vi "Main_14b.vi"() -> ()   [LabVIEW 2023]
uses:
  ENUM_Type.ctl
  <vilib>/Utility/miscctls.llb/LVMapReplaceAction.ctl
panel:
  out "Repeat index":i32
  out "Firt Index":i32
  out "Answer 2":i32
  out "Start":T1[][](array[typedef])
  in  "Puzzle":string="O.OO.#...#.O#...#...O..O.#O..O.##.....###O.O##O.O....OO.....##..##.#..O#.........O#..#..O...#O.....O\n.....###.O....#.#O.....##..O##O.......##......O..#..##.#.O#...O...O.O....#.###O.OO#.#O.#.#..O..OOO..\nOO......#.#..##O........O.###..#.#........O#..O....O#.#.##.OO.....O#.........###O......#..#.O..#....\n..#O...O....#.#.#O#....#.O#....OO.OO.O#...O##.O........O.#O.OO.O.....O.#.O.#....O.....O..OO.OO...O.#\n..#O...#.....O#O...###O......O#.##O..O#.O.O.#..#O#.O....O..O#...OO...O..#.O.......O.##OO.#...#...##.\n.#......O.OO#....O#O#OO.O..O......OOO..O....O....#OO....O...#.O.O.O..O...OOOO...#......O..#O..#O....\n..O.#.O.#..OO...........#..#......#.#...#...O...#...#...O##..O..#..O.#...O..#.O...#....#..OO..O..#.#\n.##..O..##O......#...##....#..#..O....#..##.#.O#....O#..#...O.O....O.O.........OO.#.OO......O.......\n..##O.O...O.O..O##OO..#.O..O.#...O..#..#.O...O....##...#O...O......#.....O##O#..O.#..#..O...#...#.O.\nO..##...##...#.#.OO#...OO#O..O...O.#O..#.O......O##......#O..O..OOOOOO..O.##.O...#O.....O##......OO.\n.........O..O#.....#...#......OO###OO.O.O#...#.O....O..##..O#.....O.#.##O.#......#.O.....OO#.#..##O.\nOO#O...#...OO.O####.OO.#.#.......O......O#..O#..#...#O....#.....OO#O......#O#...O#.OO......O....O#..\n.O.........#.#O#....#OO..#.........OO....O...#.O.O.O.OOO.O..O.....O.#....OOOO....OO.......#.#.O.##..\n....#.....#.O.#O...O#OO#...##.#.#..O.O.O....#O.#.#.O...#O#O.O#O...O..#OO..O###.OO..#.....OOO.#......\n#OOO..OO.O.O..O..O....#....O..O.#...O...O...##.O##..O...OOOOO#.........OOO##..#...OO#O#O.....O...##.\n.......O#..#OO.O.O..OO.O#..O.......##....OO#.O..O..O#...#..#...O.##.....#..........#.....#.O...#...O\n......O.#.O...O.......O#..O..OOO#...#........###.O..#....O.O#.OO.O..#.O#O.O.O.......O.##.OO......O.#\nO....O..........#....##.###..#...O#.O..O.##.O....O..O..O..##.O.O#OO...O.#.O##..#.#.......#.O..O..O.O\n..O#..O.#.##..O#..O#..O..O..O....OO...O##..#...O.OO..#.#.#.###O.O...#O.##..#.....#..#O.O.O...#O.O#..\n..O.##........OO.....OO.O..#.....OO.O..#...#..OOO..#....#....#.OO.#.#........OO...O.#O....##O..OOOO#\n.........#.#.OO.#O...#...O#........O..#.#........O......O#.OO..#..#....O##OO.......O..O.O.O.........\n#..O..#..OO.O.O....O..O.O.#.O.O#O...O.OO..#......OO.#..O....#.....#OOO#.OO#.OO........###....O.....O\n..O..O.O.O.....O..#.O..##.O..##..O###........O.O..#...O....OOO#.OO.#O...O..##....#.#O...#..O...O...#\nO#...O..O.#.#......O..O.#OO.....O..#.......O.##O........#O.OO..#..O.##..O.#...O...#O.....#.#..OO##..\nO.OO..O....O.#..O##O.#.O.O#O..##...O..##...#.O#.....O##.#O..O.O.....O....##..O.###......#........O..\n.....##.#.......O.OO....#..##............##..O..#.......O..O..#.O...O#..O.O.##..O..OO.O.....O...O...\n##.O.#....O..OO..OOO.OO.##..OO.OO.#...O#.....#...##...O#....OO..O.O...O...O.#....OO...#..#O#.##..#..\n........OOO....O...#.O...O..#......O....#O#.#O...O#.O........O.O...OO#....O..#.#.#O.O...OO....O.#O..\nOO...O...O..#.OO..O#.OO###..O.......#..O..O.####O....O.O.O#O.#..O..##OO..O..#....#..O#O....#..O...O.\n..O....#.O.O....O...#.........#..O#.#..OO....#...##.OO..OO.O...OOO..O..O#.###.......O#...#....OO...#\n.O...OO.O.O...#.......#.O.O.....O...OOOO.#O.O..O..OOO.OO...............#O...##O..OOO##....#O.O#.##..\nO....O...O.#...........#..#.#OO###O.O...#.O#..O.....O...O....O...#...O.OOO.OO#..OO...#..OOOO...#..#.\n....O...OO.#.O...O..#....O.O.#O..O....O..O..##O.#O....O..O.....O.......OO.......#OO#.##.O.#.O..#.##O\n#OO#.#....###O#..OO..#..O.......O.O...OO#.#O.....O.O##.O...#.##O#...O#......#..#..O#O.O.....OO.O#.O.\n...O#....O...O......#..O#O..OO.O#.OO.#.......#...O..O.....O.#O..O..O.....#OO#.O..#....#O.#O..#......\n..O.....O.......#O....O#...##.....#..O.#....#.#.#O#.#....O....#..O.O......OO....O.#OO#OO.....O......\n.#..O..#..O##...#O.#.##O#.#.#O....O#..###.OO..##..#..........O#O.#..#....O...##.......O.O.O##O#..#O.\n.#.....O..O.#..#..O....O...#.....#O.O.....OO.#..#......##........O.#.#......#...OO#....O#O.....#..O#\n#.....O.....O...O..##O.OO#OO......O#..O......O...O...#.....OO..#...O..#.....##.#.O...#..#O......OO.O\n.#..#.#.#...O#.......#.O....O..#.#.#.....O...................#.O...OOO#.....O.O.....O..O.#.....#.O.O\nO....O.....O.....O#O...O.O.O#O.#O..OO#OO..#OO.OO##.....##O#.O.O..#.....O..OO.##.#.......#...O..OO.O.\n.O#..O..#....##......O....#.#.#......#........##...#....#.......#.....O......##.#.....O.O....OO#.O..\n....OO.OO#...O..#O#O.#.O.#..OO...OOO...#O.#..#..#.#O...#O.#.O..##..O.##..O#.#.....#..O...#.O...O#.O#\n....O#....O.O#OOO...#.#.........O.O....#..O...#...#.....O.O.O.O....#.OO.##O.....#.#.#.#O..O#.O.#.OOO\nO#OO..O.#.......###..OO..O........O.##O.#O##..O...O.#OO.....#...O......O.OO...O..OO....O..O..#.#...O\n.#.O.O.O.#......O......##O...OO.....O....O#.....O#....#.......#O..#...##..O..#O.O.O..O....O.........\n...#.........OO..O.O#..O.#....#...OO##...O..OO.......#.#OO..#...#..##.#...OO#...#O.#...O.....O...#..\n#.....#O......O....O#.....#.#O.OO..........O.O...#....#.###O.O..O...#...#..#....O..O..O#.O.........#\nO.O.O...O...#.....#.#....O.O.O.....OO....#..OOO......O.O.......O#O...#.#O##O.####.........O#O.......\nO.O...........O#...OO..#O.O.O......O.......##.O...O..##...O.#OO...#OO...#...#O#.##O.#......O.##....O\nO..#...........O..O......OOO....#....OO.O...#O..O.O#......#...........#O...#O..O....#.#.#..#...#O...\n..O.....#...#...O.#.O..##.........O#..##.....#O.........................##...#.#..#.OO#O...#OOO#O.##\nOO..O.O.....O#.O....O##...O.O#.OO.#..O.....O...##.O#..O......OO..#..O.....##.....OO#OO...#O......O.O\n.OO...#....#O..#.....OO..O.O.......O#...O#..O#..#.O....#.O.#.O...O.#.O.#...#..OO.......O#....OO..O..\nO.OO..#.OOO.#.O#...#.#..O..O#.#.#.#.....#.O#..O....O..OO...O..#..#....OO#O.#......O#..##...O...O.#O.\n....#....#...OO#...O.O#OO.#.#OOO..O...OO.O..#.O#..#..O.O..#.#........OO#O.#.#.#.....OO......##.#.O..\n.#.O.OOO#OOO...##O#.#...#...##O.#...O.......###O#.##..O#..#.##...O..O.O.........O..#..O##......#.##.\nO...#..#....#O..##..O.O##..O.O###O.......O...#.O#.O#..O...#.#.O..#.....#.....O..O..OOO.OOO..O..OOO..\n...O#.O....O.O.#.O..#.O..####...OO......#OO....O#....O..O...O...OO..OO.OOO#....#..#.O.O..#..#.....O.\nO.O##O.O.O.#.O.#........#O......#O.##...##OO.......O#..#..#.O....OO........#.#O..#O.........OO.O#..O\n.......#.....O...O.O.#O##.O.OO#.....O.O#O....O.#.##.#.......##.O.O.###O...O.O#O##...#...#...O..#....\n.O#...#O...#....O##.O..........O.O.#..O.O..OOOOO.......OO.O#...O...O...#O###OOO.#OOO..............O#\nO.#.#.......OO..OO.#.O#.....#.O#O...#......O....O...O.O.....OO.#O.......#..O...O.....##OO#.....OO#.#\n...O#...#.....#..#O.#..O..O.#O#O.#...OO#O.O....O.#...#O#O....#......O..#O...#....O..O.O........#..#.\n.O.......#..O#...O....................#.##O......#.#......####..OO#...OO.##..#........#.OO..#OOO.###\n......O...O..O##.......O...O##O.O....#..#.##...#OO..##..........#..............##O.......O...#O###O.\n.........#..OO.#.......OO...O....#O.#.......O..##...###..O...#OO.O.O...#...#OO....##O.....#O.O..#...\n..#....O..O......#.#....OO#....#...O.#.OO.O#.....O#.#......O.#O.........O....O....#..O.........O....\n.OO.......#.....O.O..O#....O.#.....O..O#O...O#.....OOO....##..O.O..O#.OO...#....#...O..#..##..#..#.O\nO..#..OO##.#..OOO..#...#.OOO..O..##..O..##O.......O.O..O...#.O...#..###.#.#.#...#O..O......#.O#....#\n...O..#O..O..OO.#....#...##...O...#.......OOOO#...O.###.O.......#O.O#.##.##O..#...O...O.O..#....OO..\nOO.........OO...O.O............O....O.O...O.O.O.......O.OOO.O#....#O.O..#.....O#...#...#....#......O\n#.OO#........OO..#OO.....O.#...#..#O.O...O.....#..O.......O...O..O...O.O.O....##...O....O.OO.....#.O\n..O....#..O....O#.....#..#O......O......#...#O.......O.O...##O.#...O#..O#.#O###...#.OOO.#O...O#....O\n.#.#..OO.#..O###....O.#......O..OO...O.O..O.#.O....O.#..O.....O#....O....#.......O.O...O......OOO.#.\n...OO#.OO#O....O....O.O.#.O.#O..#.O#...###...#......#...OO##.#.#..O#...#....#.#.#.OO....O...OOOO...O\n..O.#..O...O...O#O......##.....O...O..O....#....O..#OO.#.O......#O.OOO.O.O..#........##...#O.#O...O.\n..O.OO.....O...#..O..#...O...O..#O..O#..##.....#....#.#O.#.......#O##....O.OOOOOOOO#.O...O.O#..#O##.\nO.OO.####..OO...OO.O........OO#.O.O...#....#..OO......O.O...O..#.##....O....O......#O........#O.O#..\n.#O.#...#.#...OO#.O.#O.....O##.O.OO.O..#..#O.....O...#.O.O#.....###.....#O.O.......O.#O.O#..#.O..#..\n.O......O........O...#O....##.....#O..OO.O..#.....O.#..O...#O#.#..##.#O..........O.O.O..#....#..#..#\n.OOO..O...#O.O#..#....O......O.O...O#O.....#..OO......OO.#O..O..O###......O.#.#.#.O....#...O........\n.##.....#OO#.##.....#....O..O.....OO..OO##...O...O#.##.OO#....#.......#...O.O.#.O........OO...OO....\n......OO#.....OO#OO......#.O....##..O.O#...O....#..O.O.#O.#...#.O..#.O.O#O....O.O..O.O.O.#OO.##.OO.#\n.O..OO##....O###......####.OO...O#..#..##.##.O..#..##OOO...#..#O##.#..#........#...#....O.......#.OO\n..O..O.O..#....#.#O.#.#OOO....O.##.....OO....#..O...#...#O.........O....O..#..........#.O..O.OO.O##O\nOO.......#...O#.#.......O...O.OO#.O.O.....O.....#...##..#....#.......O#.#O..O.O.......##...OO..#O...\n#O#....#.#.O..#...OO...##.#.#.O#O#...#........O..OO..#..O#..O..O.O.#O...#.....#O.#O.O#..OOO#.O.O..#.\n.#O...OO.##.#.....O...O#O................O.O..O#...#..O.#OO..O....OO...O.#...O#.#.O...O#....OO#.#...\nO#...###.OO.O...O.O#O#..O.O...O.#.....O......O...#...O.O....#...O...O#.#...##....O...........#O...#.\n.....#OO.#.OO...##.O....#OO#.....O..##...OO#.......O...##..#....#..#..##.#O.O##..O.#.O.#.O#OO.O.#.#O\nO##.#..O.OO..O.O.OOO.O...O..O.O..O.O.O..#.........#.....OO.#.......O#....#.......#O.#.O..#...O#..OOO\n.#....O.O..O##...#.OO#.O#..#OO..O.#...O....##.#O.O#O#...#.........O.#..#....OO..O.#........##O.##O..\n.....#....OO#...#.OO.O.O....O..#O.#.O#.O##.O..#.#O.#..O.#.O..O#.#.O.O.O#O....OO#...O......OO#..OO#O.\nO..O.#O..OOO..O...O...#.......#O.OO....O..#...O.....O.#.OO....#.O.OO...O#...OOO###.O..#.....O..O#.#.\n.OO......O#O.......OOO.......O..O...........O..##.....OO..##...O.O.O...O.O.O.....O..OO..O#....#.O..#\nO....#....#O.####.O...#....O....#O..#O...O.O....O.O#..O.........O#.......O....O..O...#.##..O.OO.OO..\n.O###O...#OO.OO........O.O#.O.O....O.O...##.O#..###..........#..O#.O..O.OO.O..#O#OO..O#.O.##.O.OOO##\n#.#O#..O.#...O#..#.......O#..#...#...#O..#.O.....O...O.......#O.#...#OO.O....OO..O...#.#....#O......\n..O.#O.O.O#..#.O...#.....#..O..##..O......O.OO.O.###.....#.O..O...OO#.OO.....#...OO#O..#..#O#...O..O"
  in  "Example":string="O....#....\nO.OO#....#\n.....##...\nOO.#O....O\n.O.....O#.\nO.#..O.#.#\n..O..#O..O\n.......O..\n#....###..\n#OO..#...."
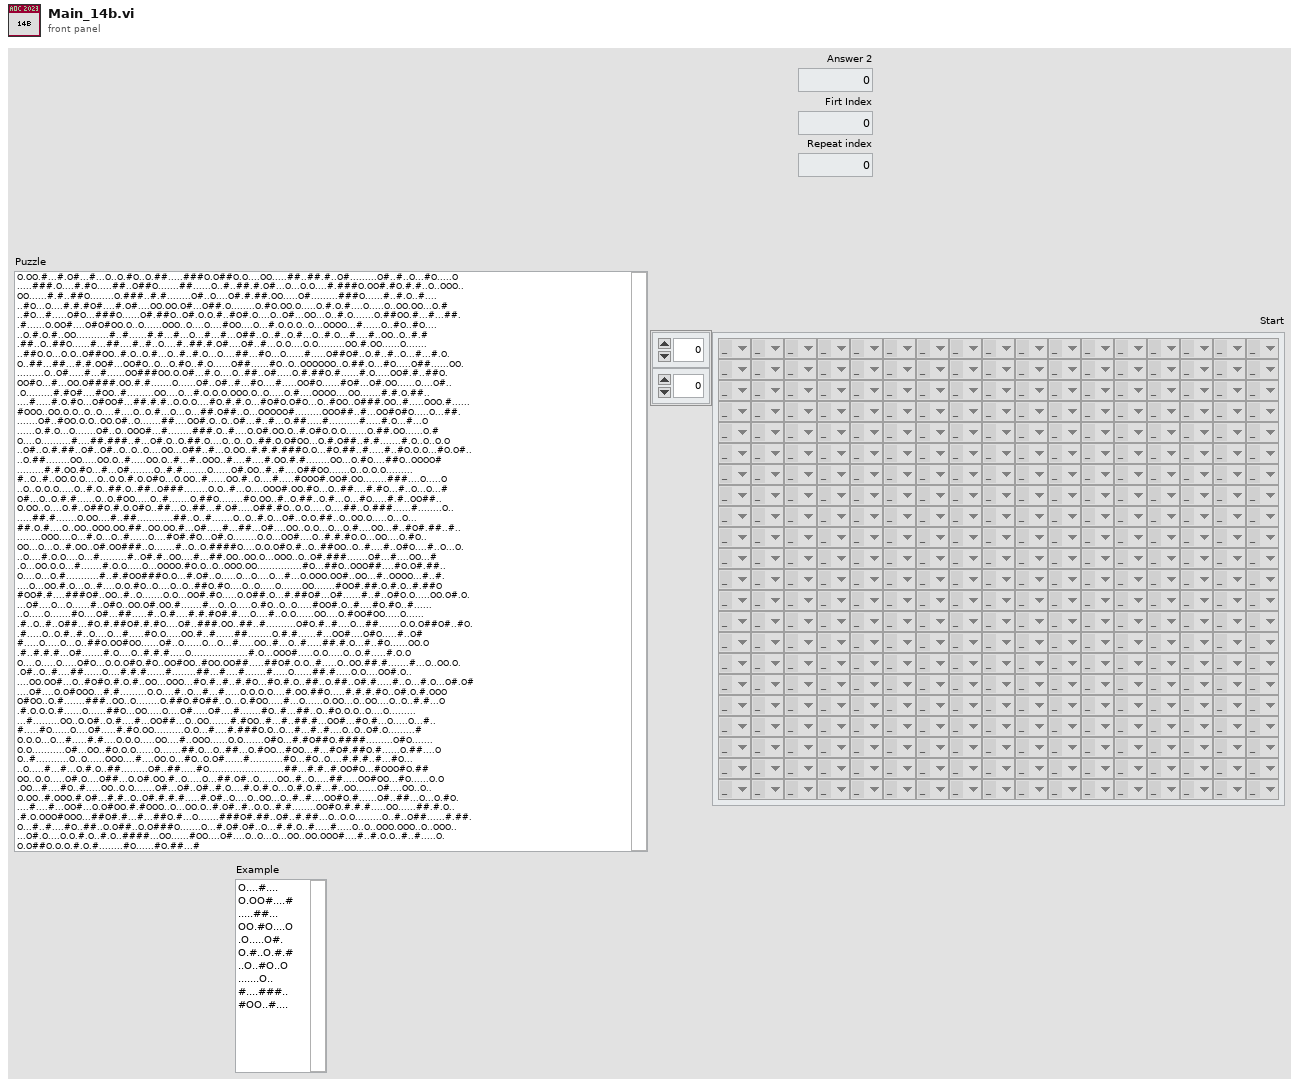
[diagram p1: front panel]
types:
  T1 = typedef "ENUM_Type.ctl" = enum16{"_", "O", "#"}
  T2 = typedef "LVMapReplaceAction.ctl" = enum32{"Modify Entry only if found", "Add or Modify Entry", "Delete Entry"}
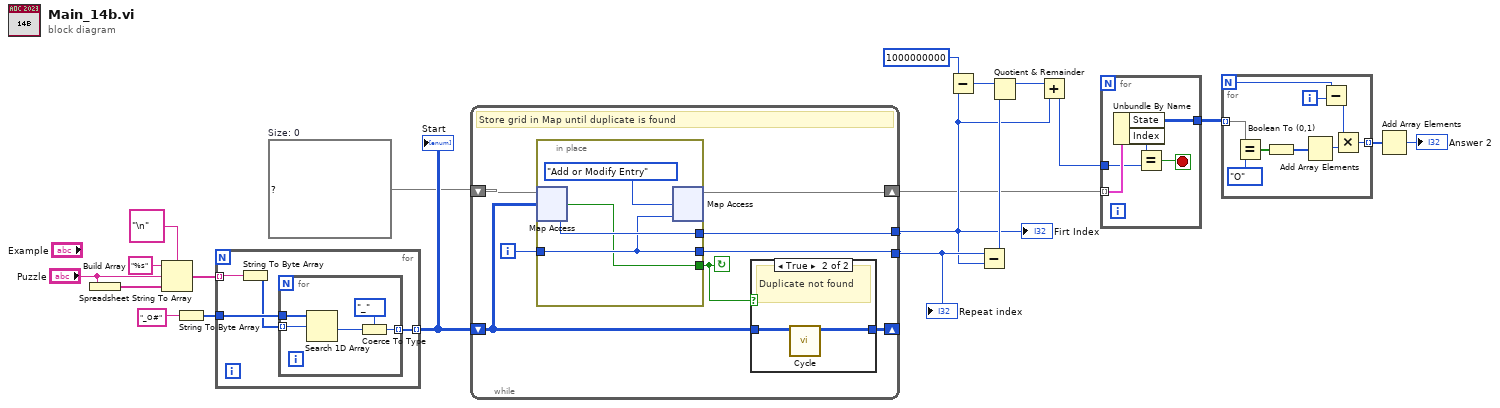
[diagram p0: block diagram]
diagram:
  w13 = map{T1[][], i32} {}  # Size: 0
  n1 = Build Array("Puzzle") -> (w20:string[])
  n2 = Spreadsheet String To Array(delimiter (Tab)="\n", format string="%s", spreadsheet string="Puzzle", array type (2D Dbl)=w20) -> (array=w17:string[])
  n3 = String To Byte Array(string="_O#") -> (unsigned byte array=w15:u8[])
  n4 = for {
    tunnel: w17 -> [w24] mode=indexing
    tunnel: w15 -> [w23]
    tunnel: [w21] -> w14 mode=indexing
    n5 = String To Byte Array(string=w24) -> (unsigned byte array=w22:u8[])
    n6 = for {
      tunnel: w23 -> [w29]
      tunnel: w22 -> [w28] mode=indexing
      tunnel: [w25] -> w21 mode=indexing
      n7 = Search 1D Array(1D array=w29, element=w28) -> (index of element=w27:i32)  [unwired: 1 in]
      n8 = Coerce To Type(0:w27, 1:ENUM_Type."_" ("Enum")) -> (2:w25:T1)
    }
  }
  "Start" <- w14
  n9 = while {
    shift-right: [w37] -> _
    shift-left: w14 -> [w35]
    shift-right: [w31] -> w6
    shift-left: w13 -> [w36]
    tunnel: [w32] -> w7
    tunnel: [w30] -> w10
    i -> [w34]
    stop <- w33 continue-if-true
    # "Store grid in Map until duplicate is found"
    n10 = in-place {
      in-place-border: w34 -> [w42]
      in-place-border: [w41] -> w33
      in-place-border: [w43] -> w32
      in-place-border: [w42] -> w30
      n11 = in-place-map #1(w36, w35) -> (w43:i32, w41:bool)  [unwired: 1 in]
      n12 = in-place-map #1(w42, LVMapReplaceAction."Add or Modify Entry" ("action")) -> (w31:map{T1[][], i32})  [unwired: 2 out]
    }
    n13 = case shown="True" w33 {
      tunnel: [w38 w40] -> w37
      tunnel: w35 -> [w38 w39]
      frame False {
        # "Duplicate Found"
      }
      frame True {
        # "Duplicate not found"
        n14 = call "Cycle.vi"("Start"=w39) -> ("Cycle array"=w40:T1[][])  [unwired: 10 in]
      }
    }
  }
  "Firt Index" <- w7
  "Repeat index" <- w10
  n15 = Subtract(x=1000000000, y=w7) -> (x-y=w11:i32)
  n16 = Subtract(x=w10, y=w7) -> (x-y=w9:i32)
  n17 = Quotient & Remainder(x=w11, y=w9) -> (x-y*floor(x/y)=w8:i32)  [unwired: 1 out]
  n18 = Add(x=w8, y=w7) -> (x+y=w5:i32)
  n19 = for {
    tunnel: w6 -> [w49] mode=indexing
    tunnel: w5 -> [w48]
    tunnel: [w45] -> w4
    stop <- w46 stop-if-true
    n20 = Unbundle By Name(w49) -> ("State"=w45:T1[][], "Index"=w47:i32)
    n21 = Equal?(x=w47, y=w48) -> (x = y?=w46:bool)
  }
  n22 = for {
    N -> [w58]
    tunnel: w4 -> [w56] mode=indexing
    tunnel: [w50] -> w2 mode=indexing
    i -> [w57]
    n23 = Equal?(x=w56, y=ENUM_Type."O" ("Enum")) -> (x = y?=w54:bool[])
    n24 = Boolean To (0,1)(Boolean=w54) -> (0, 1=w53:i16[])
    n25 = Add Array Elements(numeric array=w53) -> (sum=w52:i16)
    n26 = Subtract(x=w58, y=w57) -> (x-y=w51:i32)
    n27 = Multiply(x=w51, y=w52) -> (x*y=w50:i32)
  }
  n28 = Add Array Elements(numeric array=w2) -> (sum=→"Answer 2":i32)
